vi "Sync Project Save Config.vi"(8 "Error In":errorcluster, 10 "Project Backup Archive Directory":path, 11 "Project Source Root Directory":path) -> (0 "Error Out":errorcluster)   [LabVIEW 2011, in "LVH-Build-Tools.lvlib"]
uses:
  <vilib>/LabVIEW Hacker/Build Tools/LVH-Build-Tools.lvlib
  <vilib>/Utility/config.llb/Write Key (String).vi
  <vilib>/Utility/config.llb/NI_LVConfig.lvlib
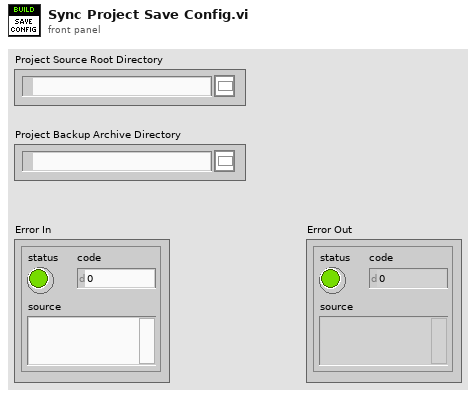
[diagram p1: front panel]
types:
  T1 = typedef "NI_LVConfig.lvlib/Config Data RefNum.ctl" = refnum<k1>
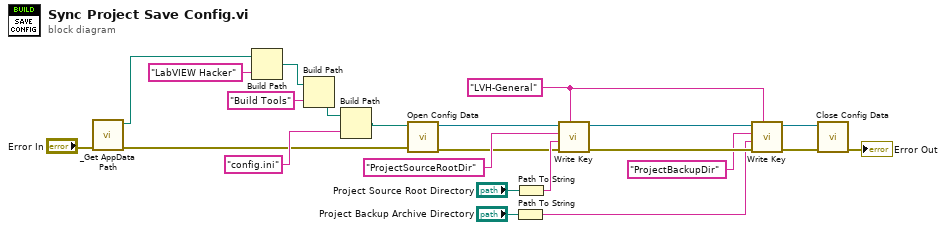
[diagram p0: block diagram]
diagram:
  w10 = "LVH-General" ("section")
  n1 = call "_Get AppData Path.vi"("Error In"="Error In") -> ("Error Out"=w2:errorcluster, "LabVIEW Data Path"=w5:path)  [unwired: 9 in]
  n2 = Build Path(base path=w5, name or relative path="LabVIEW Hacker") -> (appended path=w6:path)
  n3 = Build Path(base path=w6, name or relative path="Build Tools") -> (appended path=w4:path)
  n4 = Build Path(base path=w4, name or relative path="config.ini" ("string")) -> (appended path=w1:path)
  n5 = call <vilib>:"Open Config Data.vi"("error in (no error)"=w2, "configuration file path"=w1) -> ("error out"=w12:errorcluster, "refnum"=w11:T1)  [unwired: 7 in, 1 out]
  n6 = Path To String(path="Project Backup Archive Directory") -> (string=w18:string)
  n7 = Path To String(path="Project Source Root Directory") -> (string=w22:string)
  n8 = call-poly <vilib>:"Write Key.vi"("section"=w10, "error in (no error)"=w12, "value"=w22, "key"="ProjectSourceRootDir", "refnum"=w11) -> ("error out"=w20:errorcluster, "refnum out"=w17:T1)  [unwired: 4 in, 1 out]
  n9 = call-poly <vilib>:"Write Key.vi"("section"=w10, "error in (no error)"=w20, "value"=w18, "key"="ProjectBackupDir", "refnum"=w17) -> ("error out"=w14:errorcluster, "refnum out"=w13:T1)  [unwired: 4 in, 1 out]
  n10 = call <vilib>:"Close Config Data.vi"("error in (no error)"=w14, "refnum"=w13) -> ("error out"=→"Error Out":errorcluster)  [unwired: 8 in, 1 out]
